vi "LocalizeFromImage.vi"(0 "tracker":u64, 1 "xcor_iterations":i32=2, 2 "input image":T1) -> (6 "tracker":u64, 7 "COM":cluster{"comX":sgl, "comY":sgl}, 9 "xcorpos":cluster{"XCor X":sgl, "XCor Y":sgl}, 10 "median":sgl)   [LabVIEW 2011]
uses:
  <vilib>/vision/Image Controls.llb/IMAQ Image.ctl
  TrackerDLL.vi
panel:
  in  "XCor X":sgl
  in  "XCor Y":sgl
  in  "comX":sgl
  in  "comY":sgl
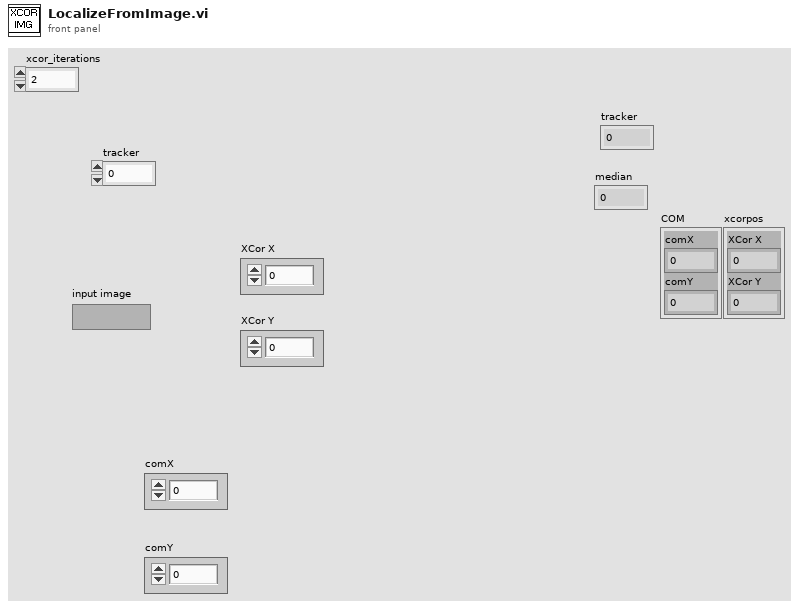
[diagram p1: front panel]
types:
  T1 = typedef "IMAQ Image.ctl" = refnum<image>
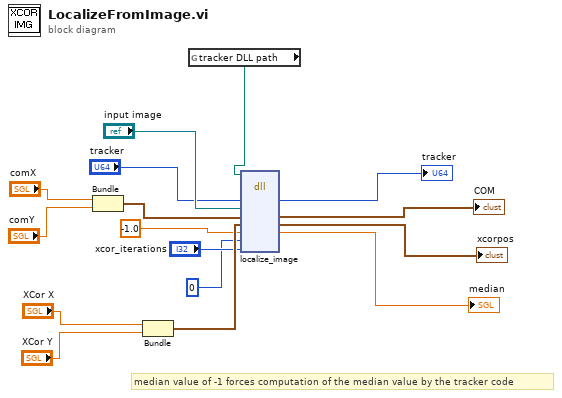
[diagram p0: block diagram]
diagram:
  # "median value of -1 forces computation of the median value by the tracker code"
  n1 = Bundle("comX"="comX", "comY"="comY") -> (w14:cluster{"comX":sgl, "comY":sgl})  [unwired: 1 in]
  n2 = Bundle("XCor X"="XCor X", "XCor Y"="XCor Y") -> (w11:cluster{"XCor X":sgl, "XCor Y":sgl})  [unwired: 1 in]
  n3 = global read "TrackerDLL.vi" "tracker DLL path"() -> (w5:path)
  n4 = dll-call lib="D:/jcnossen1/cudaqi-tracker/Debug/cputrack.dll" fn="localize_image"(path in=w5, "tracker"="tracker", "image"="input image", "COM"=w14, "xcorpos"=w11, "median"=sgl -1.0, "debugImage"=u64 0, "xcor_iterations"="xcor_iterations") -> ("tracker"=→"tracker":u64, "COM"=→"COM":cluster{"comX":sgl, "comY":sgl}, "xcorpos"=→"xcorpos":cluster{"XCor X":sgl, "XCor Y":sgl}, "median"=→"median":sgl)  [unwired: 6 in, 2 out]
